vi "Observe Data.vi"(6 "Time Stamp":timestamp, 8 "error in (no error)":errorcluster, 9 "Value":variant, 10 "Datum Name":string, 11 "IObserver in":refnum<class "IObserver.lvclass">) -> (0 "error out":errorcluster, 3 "IObserver out":refnum<class "IObserver.lvclass">)   [LabVIEW 2015, in "IObserver.lvlib" / "IObserver.lvclass"]
doc: "<License>\nCopyright © 2017 Composed Systems, LLC | All rights reserved\nwww.composed.io\n\nAuthor: Ethan Stern <ethan.stern@composed.io>\n\nThis software is provided \"AS IS\" WITHOUT WARRANTIES, either express or implied, AND IS FOR EDUCATIONAL PURPOSES ONLY.\n</License>"
uses:
  IObserver.lvclass
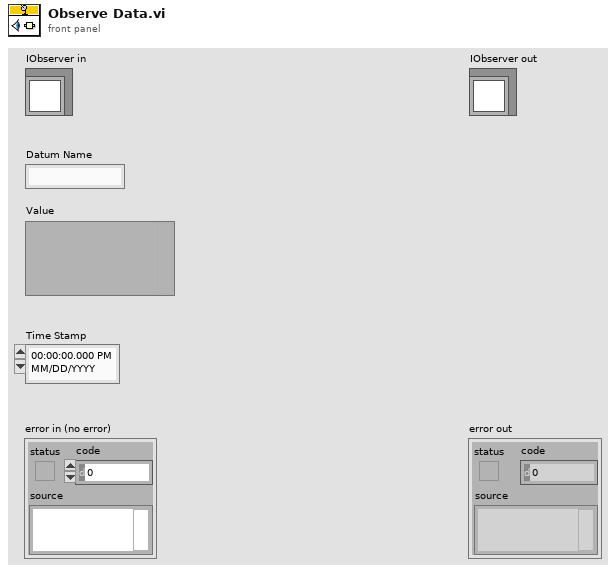
[diagram p1: front panel]
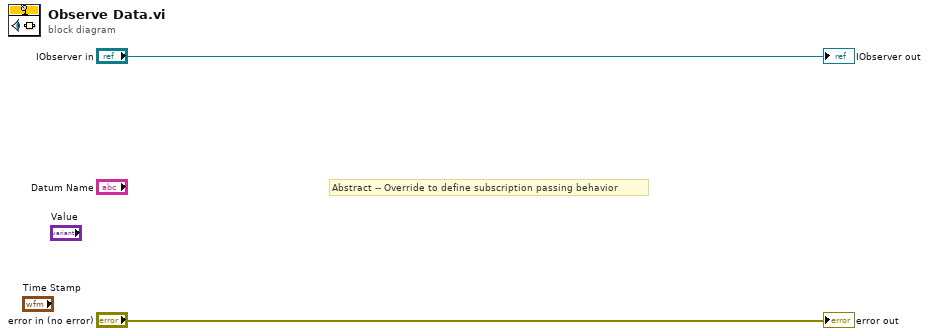
[diagram p0: block diagram]
diagram:
  # "Abstract -- Override to define subscription passing behavior"
  "error out" <- "error in (no error)"
  "IObserver out" <- "IObserver in"
